vi "gen_axis_data.vi"(7 "size":i32, 10 "step":dbl, 11 "start":dbl) -> (3 "Array":dbl[](array[numeric]))   [LabVIEW 2021]
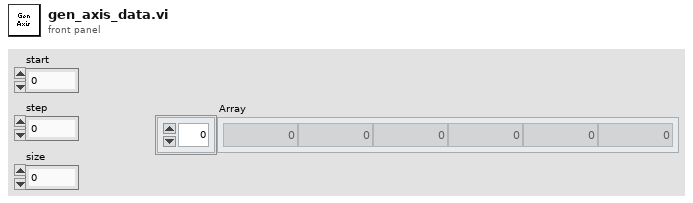
[diagram p1: front panel]
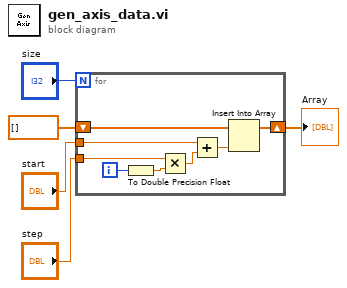
[diagram p0: block diagram]
diagram:
  n1 = for {
    N: "size" -> [_]
    shift-right: [w6] -> w1
    shift-left: dbl[] [] -> [w13]
    tunnel: "step" -> [w10]
    tunnel: "start" -> [w8]
    i -> [w11]
    n2 = To Double Precision Float(number=w11) -> (double precision float=w9:dbl)
    n3 = Multiply(x=w10, y=w9) -> (x*y=w12:dbl)
    n4 = Add(x=w8, y=w12) -> (x+y=w7:dbl)
    n5 = Insert Into Array(array=w13, new element=w7) -> (w6:dbl[])  [unwired: 1 in]
  }
  "Array" <- w1
